vi "Convert Boolen to Digital Waveform LV2016 NI Verified.vi"() -> ()   [LabVIEW 2016]
uses:
  <vilib>/Waveform/DWDTOps.llb/DWDT Boolean Array to Digital.vi
panel:
  in  "Boolean":bool=TRUE
  out "appended array":bool[](array[boolean])
  out "Digital Waveform Graph":digitalwaveform(graph)
  # "Overview: This VI demonstrates how you can take a boolean input, and convert it to a Digital Waveform in LabVIEW.\nRequirements:\nLabVIEW 2012 (or compatible)\nInstructions:\nRun this VI"
  # "Run the VI and you will\nnote that the boolean \nabove creates an array\nof 01010 that it then \nwrites out as a digital \nwaveform"
  # "Setting the boolean\nto True, negates the\ninput, making the output\n10101"
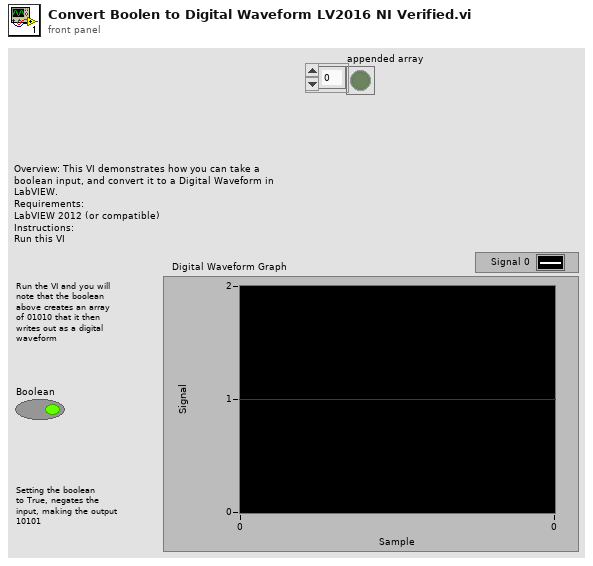
[diagram p1: front panel]
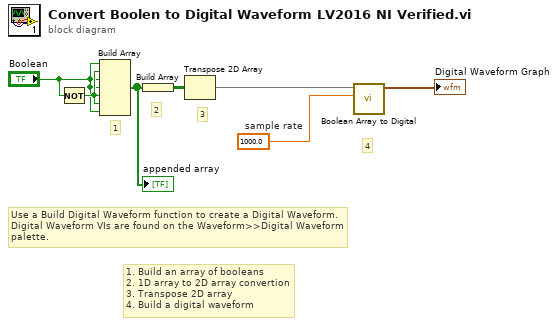
[diagram p0: block diagram]
diagram:
  w5 = 1000.0  # sample rate
  # "1. Build an array of booleans\n2. 1D array to 2D array convertion\n3. Transpose 2D array\n4. Build a digital waveform"
  # "4"
  # "3"
  # "2"
  # "1"
  # "Use a Build Digital Waveform function to create a Digital Waveform.\nDigital Waveform VIs are found on the Waveform>>Digital Waveform\npalette."
  n1 = Not(x="Boolean") -> (.not. x?=w2:bool)
  n2 = Build Array("Boolean", w2, "Boolean", "Boolean", w2, w2, "Boolean") -> (w6:bool[])
  "appended array" <- w6
  n3 = Build Array(w6) -> (w4:bool[][])
  n4 = Transpose 2D Array(2D array=w4) -> (transposed array=w3:bool[][])
  n5 = call-poly <vilib>:"Boolean Array to Digital.vi"("sample rate"=w5, "boolean array"=w3) -> ("digital waveform"=→"Digital Waveform Graph":digitalwaveform)  [unwired: 3 in, 6 out]
